vi "DiffDrivePoseEst2_Pack_Config.vi"(5 "TrackWidth_Meters":dbl=1.2, 6 "Vision Heading std dev Rad":dbl=0.05, 7 "Odom X std dev M":dbl=0.02, 8 "Vision Y std dev M":dbl=0.1, 9 "Vision X std dev M":dbl=0.1, 10 "Odom Heading std dev Rad":dbl=0.01, 11 "Odom Y std dev M":dbl=0.02) -> (3 "DiffPoseEst2Config":T1={"TrackWidth_Meters"=1.2, "Odom X std dev M"=0.02, "Odom Y std dev M"=0.02, "Odom Heading std dev Rad"=0.01, "Vision X std dev M"=0.1, "Vision Y std dev M"=0.1, "Vision Heading std dev Rad"=0.05} {"Vision Heading std dev Rad" format="%#_13g"; "Vision Y std dev M" format="%#_13g"; "Vision X std dev M" format="%#_13g"; "Odom Heading std dev Rad" format="%#_13g"; "Odom Y std dev M" format="%#_13g"; "Odom X std dev M" format="%#_13g"; "TrackWidth_Meters" format="%#_13g"})   [LabVIEW 2019, in "Trajectory_Library.lvlib"]
doc: "Pack indvidual values into the cluster required by the DiffDrivePoseEst2_Execute function. \n\nInputs\n - TrackWidth_Meters -- double -- Effective tract width (meters)\n - Odom X Std Dev M -- double -- Odometry X position standard deviation (Default: 0.02) (meters)\n - Odom Y Std Dev M -- double -- Odometry Y position standard deviation (Default: 0.02) (meters)\n - Odom Heading Std Dev M -- double -- Odometry Heading (gyro) position standard deviation (Default: 0.01) (radians)\n - Vision X Std Dev M -- double -- Vision X position standard deviation (Default: 0.1) (meters)\n - Vision Y Std Dev M -- double -- Vision Y position standard deviation (Default: 0.1) (meters)\n - Vision Heading Std Dev M -- double -- Vision Heading (gyro) position standard deviation (Default: 0.05) (radians)\n\nOutputs:\n - DiffPoseEst2Config -- cluster -- Packed data values."
uses:
  Trajectory_Library.lvlib
  TypeDef/DIFF_DRIVE_POSE_EST2_CONFIG.ctl
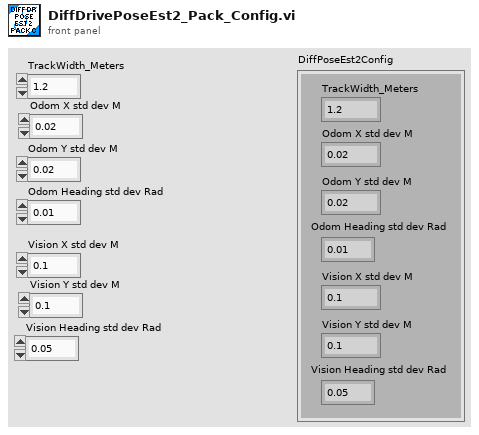
[diagram p1: front panel]
types:
  T1 = typedef "Trajectory_Library.lvlib/DIFF_DRIVE_POSE_EST2_CONFIG.ctl" = cluster{"TrackWidth_Meters":dbl, "Odom X std dev M":dbl, "Odom Y std dev M":dbl, "Odom Heading std dev Rad":dbl, "Vision X std dev M":dbl, "Vision Y std dev M":dbl, "Vision Heading std dev Rad":dbl}
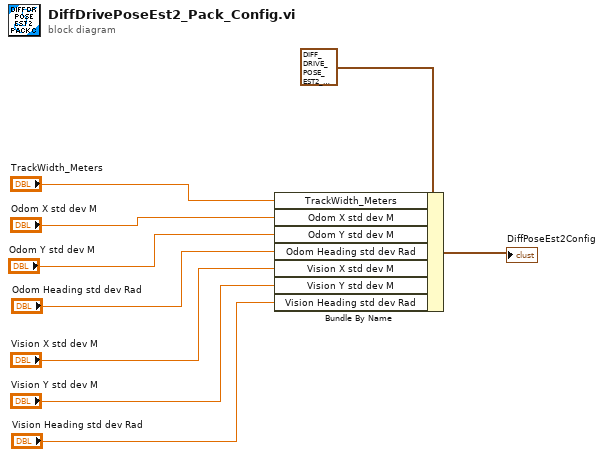
[diagram p0: block diagram]
diagram:
  n1 = Bundle By Name(cluster=T1 {"TrackWidth_Meters"=1.2, "Odom X std dev M"=0.02, "Odom Y std dev M"=0.02, "Odom Heading std dev Rad"=0.01, "Vision X std dev M"=0.1, "Vision Y std dev M"=0.1, "Vision Heading std dev Rad"=0.05} ("DiffPoseEst2Config"), "TrackWidth_Meters"="TrackWidth_Meters", "Odom X std dev M"="Odom X std dev M", "Odom Y std dev M"="Odom Y std dev M", "Odom Heading std dev Rad"="Odom Heading std dev Rad", "Vision X std dev M"="Vision X std dev M", "Vision Y std dev M"="Vision Y std dev M", "Vision Heading std dev Rad"="Vision Heading std dev Rad") -> (→"DiffPoseEst2Config":T1)
